vi "Temperature2(Post).vi"(7 "LabVIEW Web Service Request":refnum<class "Web Request.lvclass">) -> ()   [LabVIEW 2019]
uses:
  <vilib>/wsapi/Web Request.lvclass
  QDMH support files/QDMH Poly VIs/QDMH POLY Enqueue Cluster.vi
panel:
  # "Use the Web Service Request input terminal to call the VIs on the Web Services palette. Do not remove it from the connector pane unless you don't need access to the palette."
  # "Each additional control wired to the connector pane will be available as an input in the URL. To include an indicator in terminal-mode output (the default setting), it must also be wired to the connector pane."
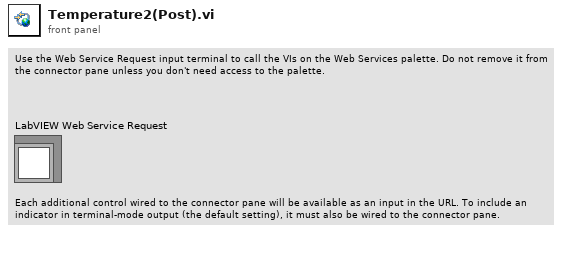
[diagram p1: front panel]
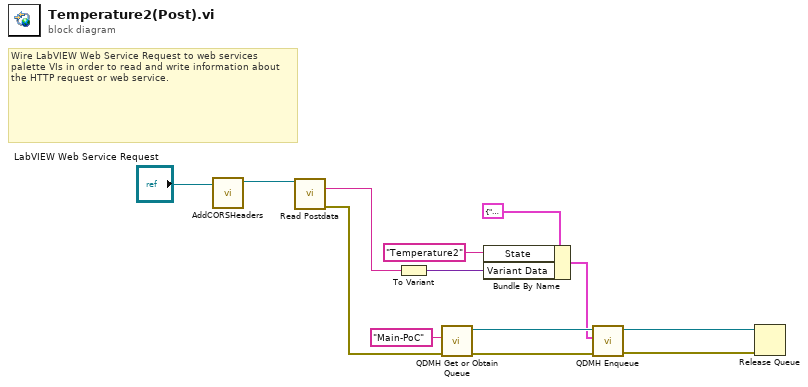
[diagram p0: block diagram]
diagram:
  # "Wire LabVIEW Web Service Request to web services palette VIs in order to read and write information about the HTTP request or web service."
  n1 = call "AddCORSHeaders.vi"("Web Request in"="LabVIEW Web Service Request") -> ("Web Request out"=w13:refnum<class "Web Request.lvclass">)  [unwired: 10 in]
  n2 = call <vilib>:"Read Postdata.vi"("LabVIEW Web Service Request"=w13) -> ("postdata"=w6:string, "error out"=w9:errorcluster)  [unwired: 12 in, 1 out]
  n3 = To Variant(anything=w6) -> (Variant=w5:variant)
  n4 = call "QDMH Get or Obtain Queue.vi"("error in (no error)"=w9, "Queue Name"="Main-PoC") -> ("error out"=w10:errorcluster, "queue out"=w11:refnum<queue>)  [unwired: 1 in, 7 out]
  n5 = Bundle By Name(cluster=cluster{"State":string, "Variant Data":variant} {"State"="", "Variant Data"=variant} ("QDSM Element"), "State"="Temperature2", "Variant Data"=w5) -> (w4:cluster{"State":string, "Variant Data":variant})
  n6 = call-poly "QDMH Enqueue.vi"("error in (no error)"=w10, "QDSM Element"=w4, "queue"=w11) -> ("error out"=w2:errorcluster, "queue out"=w3:refnum<queue>)  [unwired: 7 out]
  n7 = Release Queue(queue=w3, error in (no error)=w2) -> ()  [unwired: 1 in, 3 out]
